vi "Read Hardware.vi"(8 "error in (no error)":errorcluster, 11 "Instrument in":refnum<class "Instrument.lvclass">) -> (0 "error out":errorcluster, 2 "response":string, 3 "Instrument out":refnum<class "Instrument.lvclass">)   [LabVIEW 2019, in "Instrument.lvlib" / "Instrument.lvclass"]
doc: "Override <b>Read Hardware</b> to write to your instrument hardware."
uses:
  Instrument.lvclass
  Instrument.lvclass/Instrument.ctl
  subsystems/HAL/HAL.lvclass
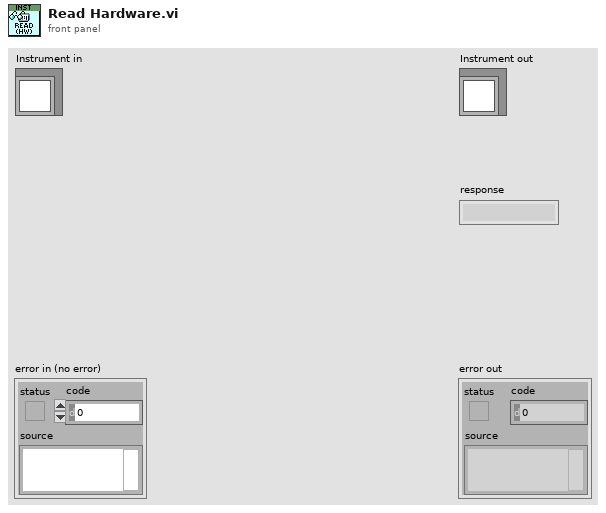
[diagram p1: front panel]
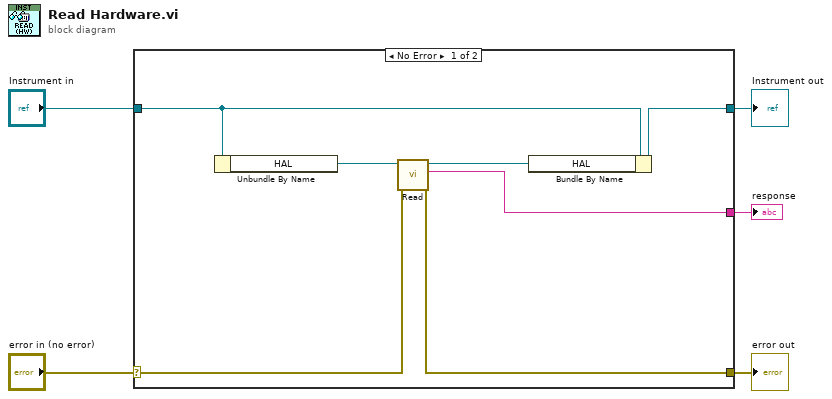
[diagram p0: block diagram]
diagram:
  n1 = case shown="No Error" "error in (no error)" {
    selector: "error in (no error)" -> [w8 w14]
    tunnel: [w7 w14] -> w4
    tunnel: [w11 w13] -> w2
    tunnel: "Instrument in" -> [w10 w13]
    tunnel: [w6 _] -> w1
    frame No Error {
      n2 = Unbundle By Name(w10) -> ("HAL"=w12:refnum<class "HAL.lvclass">)
      n3 = call-dynamic "Read.vi"("error in (no error)"=w8, "HAL in"=w12) -> ("error out"=w7:errorcluster, "response"=w6:string, "HAL out"=w9:refnum<class "HAL.lvclass">)  [unwired: 7 in]
      n4 = Bundle By Name(cluster=w10, "HAL"=w9) -> (w11:refnum<class "Instrument.lvclass">)
    }
    frame Error {
    }
  }
  "error out" <- w4
  "Instrument out" <- w2
  "response" <- w1
